vi "traceFileIO_readFromFile.vi"(0 "reference":refnum<class "OSA.lvclass">, 1 "path":path, 3 "dataType":T1, 4 "trace idx":u32, 5 "error in (no error)":errorcluster, 7 "dialog (empty path)":bool) -> (14 "duplicate reference":refnum<class "OSA.lvclass">, 17 "cancelled":bool, 19 "error out":errorcluster)   [LabVIEW 2010, in "OSA.lvclass"]
doc: "Reads trace data from spf2 binary file and store into trace buffer."
uses:
  OSA.lvclass
  typeDef/trace_properties_ui.ctl
  typeDef/acq_dataType.ctl
  OSA20X_misc.lvlib
  FTSLib.dll
panel:
  in  "property":T2=enum."type"
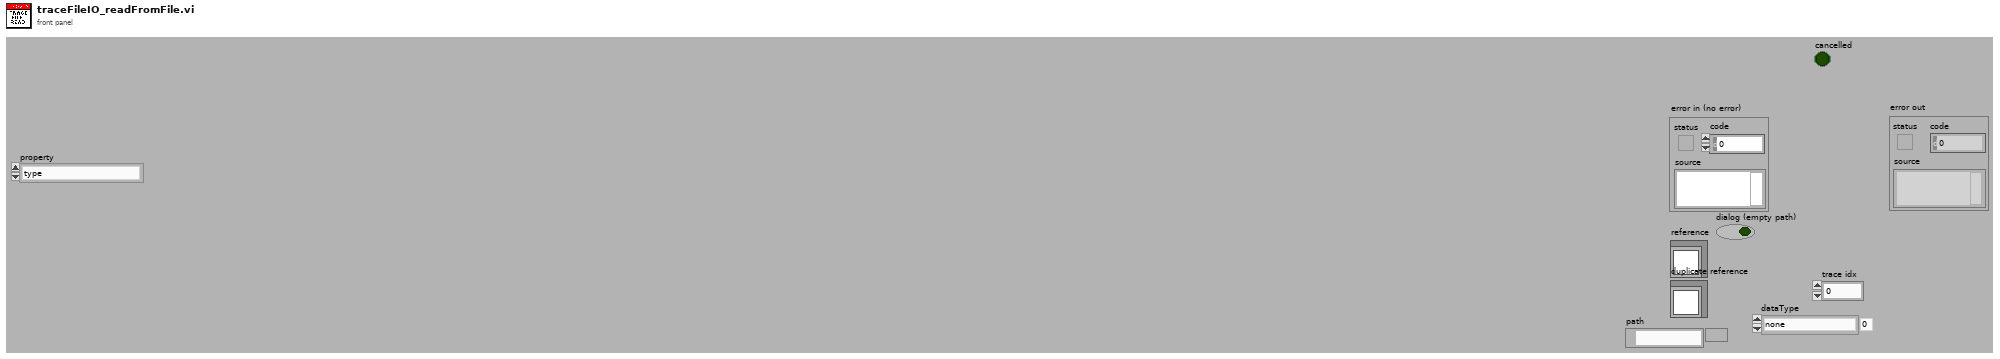
[diagram p1: front panel]
types:
  T1 = typedef "OSA.lvclass/acq_dataType.ctl" = enum16{"none", "interferogram", "spectrum"}
  T2 = typedef "OSA.lvclass/trace_properties_ui.ctl" = enum16{"length", "type", "acquisitionMode", "xValueFormat", "date", "time", "averageNum", "smoothType", "igramSmoothType", "phaseCorrection", "apodisation", "__allocatedLengthI", "__allocatedLengthx", "adcBits", "sensitivityMode", "resolutionMode", "rollingAverage", "samplesPerReference", "air_measureOption", "interferogramProperty", "all_uiProperties"}
  T3 = enum16{"length", "type", "acquisitionMode", "xValueFormat", "date", "time", "averageNum", "smoothType", "igramSmoothType", "phaseCorrection", "apodisation", "__allocatedLengthI", "__allocatedLengthx", "adcBits", "sensitivityMode", "resolutionMode", "rollingAverage", "samplesPerReference", "air_measureOption", "interferogramProperty", "all_uiProperties"}
  T4 = typedef "OSA.lvclass/ObjectAttributes.ctl" = cluster{"Stop":bool, "dataType":T1, "spectrometerIdx":u16, "buffer size interferogram":i32, "interferogram":cluster{"new":bool, "plot_x_ min":sgl, "plot_x_max":sgl, "plot_y_min":sgl, "plot_y_max":sgl, "Graph Intrfrgrm":T5, "timeStamp":u32, "signal (%)":dbl, "traces":cluster{"idx":u32, "broadBand":bool, "monoChromatic":bool, "peakToPeakSignal":dbl, "peakToPeakPos":dbl}[], "traces idx last":i32}, "spectrum":cluster{"new":bool, "plot_x_min":sgl, "plot_x_max":sgl, "plot_unit_x":T6, "plot_unit_y":T7, "plot_y_min":sgl, "plot_y_max":sgl, "Graph Spectrum":T5, "timeStamp":u32, "X_VAL_OPTIONS":enum16{"MIN_MAX", "ARRAY"}, "traces":cluster{"idx":u32}[], "traces idx last":i32}, "Thorlabs_OSA_64.lvclass:queue_action.ctlqueue ref":refnum<queue>, "action":T8, "plot zoom step":dbl, "buffer semaphore":T9, "acq stopped":bool, "dataType active":T1, "temperature (degr C)":sgl, "pressure (hPa)":sgl, "rel humidity (%)":sgl, "settings":cluster{"resolution":u16, "sensitivity":u16, "Average":bool, "average nr":u32, "apodisation":T10, "acq delay (ms)":u32, "airMesure":T11, "wmtr on":bool, "intfgrm_smooth_width":u16, "intfgrm_smooth_nrOfPasses":u16, "intfgrm_smooth":T12, "phaseCorrection":T13, "zeroFill":u8, "spectr_smooth":T12, "spectr_smooth_width":u16, "spectr_smooth_nrOfPasses":u16, "resolution (/cm)":sgl, "REF wavelength, (nm)":dbl, "gain_idx":u16, "gainAuto":bool, "gain_relative":dbl, "PD sensitivity mode":T14, "PD senseMode implemented":bool, "SensorTemperature implemented":bool, "SensorPressure implemented":bool, "SensorHumidity implemented":bool}, "peaks position":sgl[], "peaks width":sgl[], "peaks height":sgl[], "peaks max nr":u32, "peaks latest nr":i32, "peaks new":bool, "power":dbl, "power new":bool, "path":string, "wavelength (WNr)":dbl, "wavelength new":bool, "buffer size spectrum":i32, "status":string, "VI reference":refnum<vi>, "funcPointer":u64, "libraryPointer":u64, "singleAcquisition":bool, "coherenceLength (cm)":dbl, "coherenceLength new":bool, "spectrometer model":string, "spectrometer serial nr":string, "peaks thld left":sgl[], "peaks thld right":sgl[], "coherenceLength error (cm)":dbl, "ADC bits":u16, "peaks position centroid":sgl[], "peaks height centroid":sgl[], "OSA series":T15, "channel index spectrum":u16, "spectrometer rangeLow, (/cm)":dbl, "spectrometer rangeHigh, (/cm)":dbl, "channel index interferogram":u16}
  T5 = typedef "OSA.lvclass/graph_intensity.ctl" = refnum<vi>
  T6 = typedef "OSA.lvclass/spectrum_x_unit.ctl" = enum16{"wavenr/cm", "THz", "eV", "nm_air", "nm_vac"}
  T7 = typedef "OSA.lvclass/y_unit.ctl" = enum16{"ADC counts", "dBm pwr absolute", "dBm pwr density", "mW pwr absolute", "mW pwr density"}
  T8 = typedef "OSA.lvclass/queue_action.ctl" = enum16{"none", "stop", "GUI_plotInterferogram", "GUI_plotSpectrum", "GUI_plotInterferogramRescale", "GUI_plotSpectrumRescale", "GUI_plotInterferogramReset", "GUI_plotSpectrumReset", "GUI_plotInterferogramAutoScaleY", "GUI_plotSpectrumAutoScaleY", "GUI_plotInterferogramZoomOut", "GUI_plotSpectrumZoomOut", "GUI_plotInterferogramPane", "GUI_plotSpectrumPane", "GUI_plotInterferogramZoomMouse", "GUI_plotSpectrumZoomMouse", "ENVIRONMENT temperature", "ENVIRONMENT pressure", "MODE_resolution set", "MODE_resolution get", "MODE_sensitivity set", "MODE_sensitivity get", "MODE_PDTemperature set", "MODE_PDTemperature get", "REBOOT/RESET firmware", "ACQASYNC_acquireSingleSpectrum", "ACQASYNC_continuous start", "ACQASYNC_continuous stop\n", "ACQASYNC_get last interferogram", "ACQASYNC_get last spectrum", "ACQASYNC_get last waveNr", "ACQOPT_interferogram smoothing set", "ACQOPT_interferogram smoothing get", "ACQOPT_spectrum smoothing set", "ACQOPT_spectrum smoothing get", "ACQOPT_apodisation type set", "ACQOPT_apodisation type get", "ACQOPT_phase correction type set", "ACQOPT_phase correction type get", "ACQOPT_acqIntervall_set", "ACQOPT_acqIntervall_get", "ACQOPT_average spectrum set", "ACQOPT_average spectrum get", "ACQOPT_rolling average set", "ACQOPT_rolling average get", "ACQOPT_zero fill factor set", "ACQOPT_zero fill factor get", "ACQOPT_cycle counting set", "ACQOPT_cycle counting get", "ACQOPT_air measure option set", "ACQOPT_air measure option get", "ACQOPT_gainLevel auto get", "ACQOPT_gainLevel auto set", "ACQOPT_gainLevel get", "ACQOPT_gainLevel set", "ACQOPT_getAll", "INSTRUMENT_PROPERTY_range_WaveNr_min", "INSTRUMENT_PROPERTY_range_WaveNr_max", "INSTRUMENT_PROPERTY_reference_wavelength_cm^-1", "INSTRUMENT_PROPERTY_samplesPerRefPeriod", "INSTRUMENT_PROPERTY_resolution_waveNrPercm", "INSTRUMENT_PROPERTY_availableGainLevels", "INSTRUMENT_PROPERTY_status", "CONVERT", "ANALYSE_POWER", "ANALYSE_PEAKS", "ANALYSE_WAVELENGTH", "ANALYSE_SPECTRUM", "ANALYSE_INTERFEROGRAM", "ANALYSE_COHERENCE_LENGTH", "MATH", "MATH_power", "MATH_peaks", "FILE", "miscellaneous"}
  T9 = typedef "Semaphore RefNum" = refnum<k1>
  T10 = typedef "OSA.lvclass/apodisation.ctl" = enum16{"NONE", "NORTON_BEER_WEAK", "NORTON_BEER_MEDIUM", "NORTON_BEER_STRONG", "TRIANGULAR", "COSINE", "HANN", "HAMMING", "BLACKMANHARRIS3", "BLACKMANHARRIS4", "GAUSSIAN"}
  T11 = typedef "OSA.lvclass/airMeasure.ctl" = enum16{"TEMPERATURE", "PRESSURE"}
  T12 = typedef "OSA20X_misc.lvlib/interferogram_smoothing.ctl" = enum16{"NONE", "BINOMIAL", "SAVITSKY_GOLAY", "FOURIER", "MOVING_AVERAGE", "GAUSSIAN"}
  T13 = typedef "OSA.lvclass/phaseCorrection.ctl" = enum16{"NONE", "MERTZ", "FORMAN", "MERTZ_FILE", "FORMAN_FILE", "FUTURE COMP."}
  T14 = typedef "OSA20X_misc.lvlib/PDTemperatureMode.ctl" = enum16{"cool: better sensitivity/noise floor", "warm: extended wl range"}
  T15 = typedef "OSA.lvclass/OSA_series.ctl" = enum16{"OSA200", "OSA300", "UNKNOWN"}
  T16 = cluster{"idx":u32, "broadBand":bool, "monoChromatic":bool, "peakToPeakSignal":dbl, "peakToPeakPos":dbl}[]
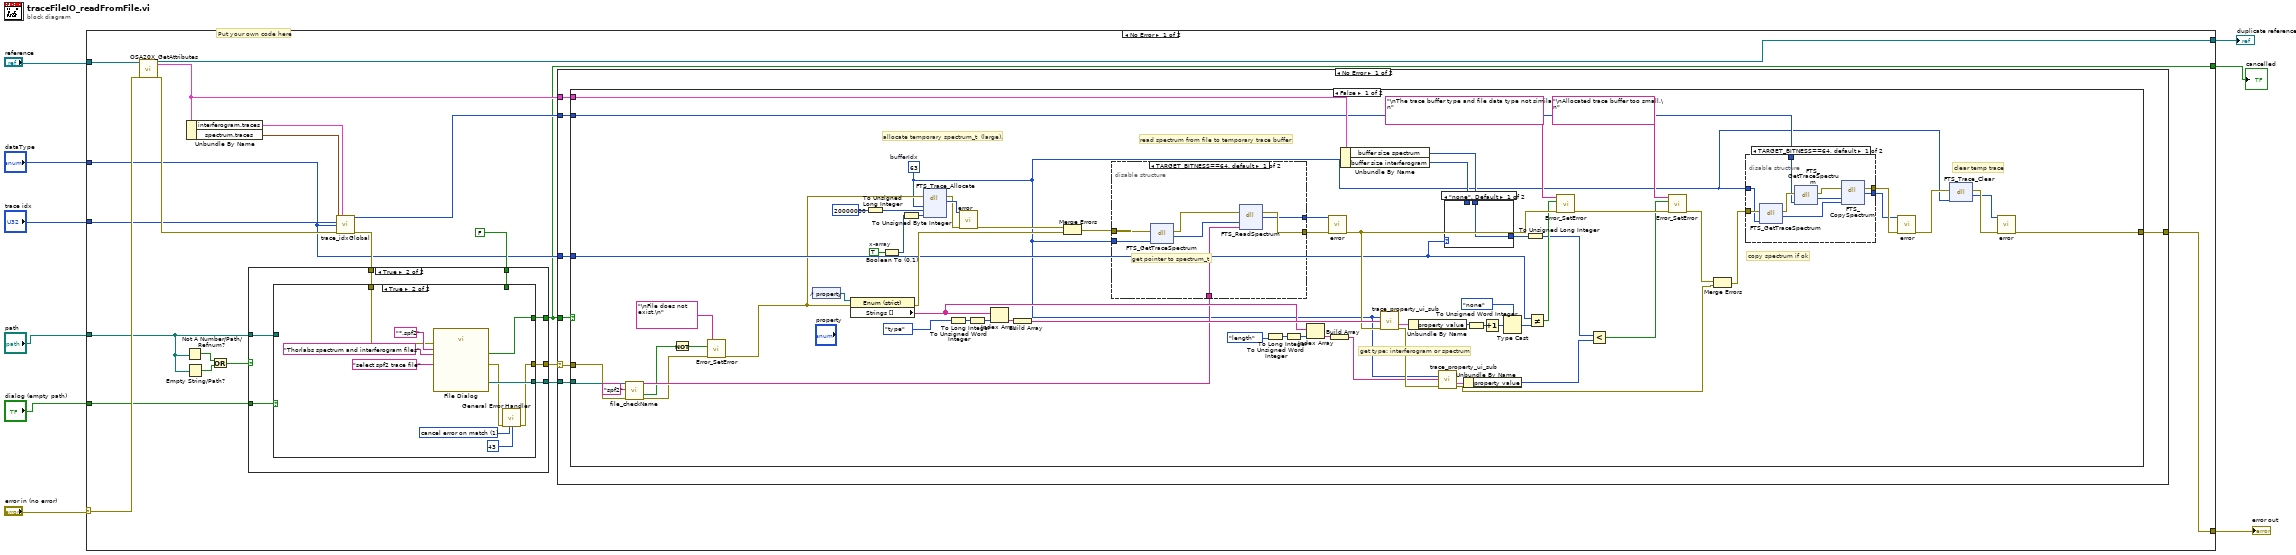
[diagram p0: block diagram]
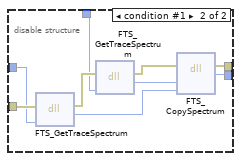
[diagram p2: hidden frame]
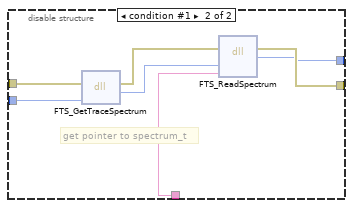
[diagram p4: hidden frame]
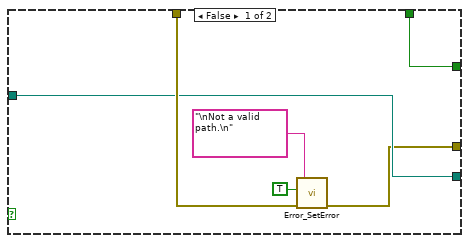
[diagram p8: hidden frame]
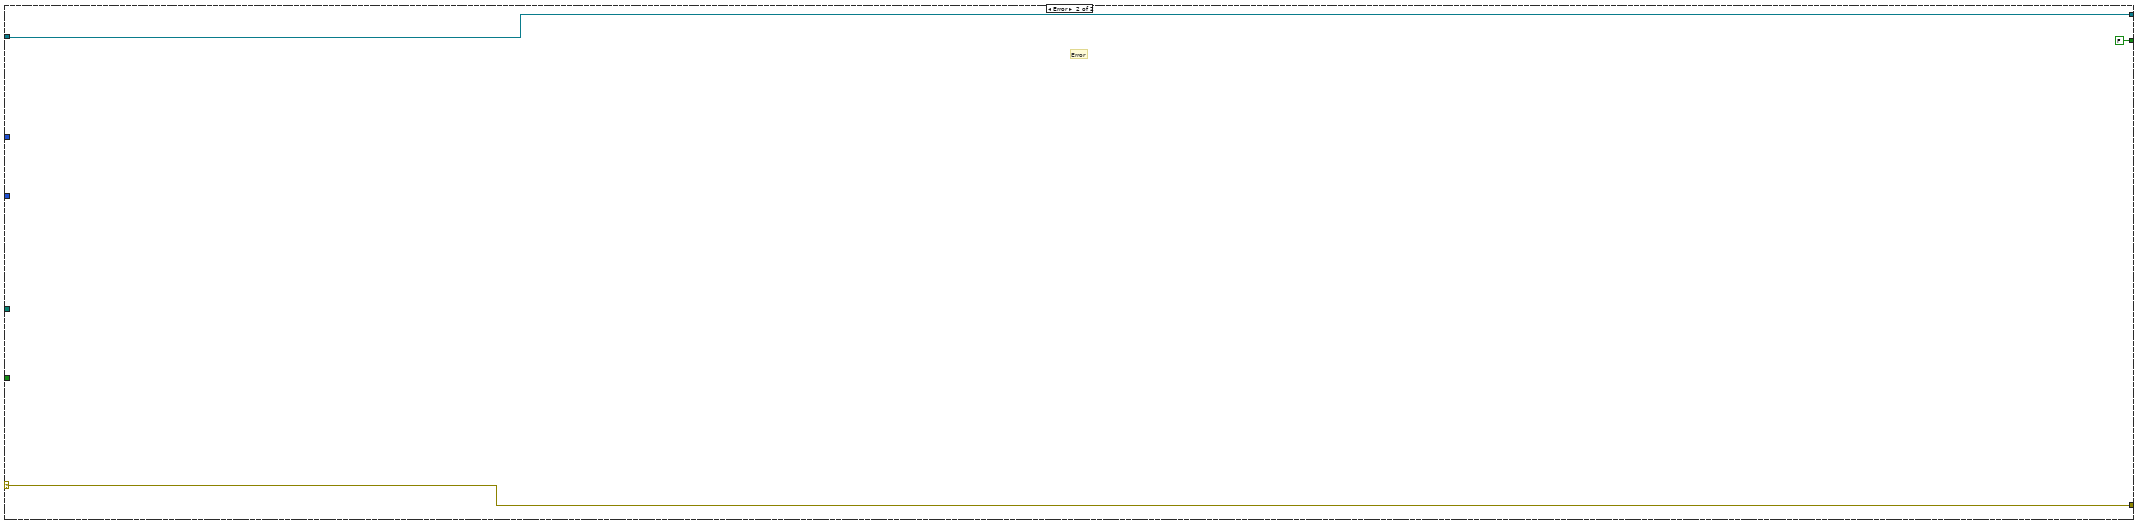
[diagram p9: hidden frame]
diagram:
  n1 = case shown="No Error" "error in (no error)" {
    selector: "error in (no error)" -> [w29 w167]
    tunnel: [w19 w167] -> w8
    tunnel: "reference" -> [w30 w166]
    tunnel: [w20 w166] -> w6
    tunnel: "trace idx" -> [w13 _]
    tunnel: "path" -> [w14 _]
    tunnel: "dataType" -> [w12 _]
    tunnel: "dialog (empty path)" -> [w11 _]
    tunnel: [w10 FALSE ("cancelled")] -> w1
    frame No Error {
      # "Put your own code here"
      n2 = call "OSA20X_GetAttributes.vi"("reference in"=w30, "error in (no error)"=w29) -> ("reference out"=w20:refnum<class "OSA.lvclass">, "Data"=w16:T4, "error out"=w15:errorcluster)  [unwired: 14 in, 1 out]
      n3 = Not A Number/Path/Refnum?(number/path/refnum=w14) -> (NaN/Path/Refnum?=w27:bool)
      n4 = Empty String/Path?(string/path=w14) -> (empty?=w28:bool)
      n5 = Unbundle By Name(w16) -> ("interferogram.traces"=w18:T16, "spectrum.traces"=w17:cluster{"idx":u32}[])
      n6 = Or(x=w27, y=w28) -> (x .or. y?=w26:bool)
      n7 = call "trace_idxGlobal.vi"("traces_spectrum"=w17, "traces_interferogram"=w18, "trace idx"=w13, "dataType"=w12, "error in (no error)"=w15) -> ("global trace idx"=w25:u32, "error out"=w24:errorcluster)  [unwired: 9 in]
      n8 = case shown="True" w26 {
        tunnel: w14 -> [w140 w144]
        tunnel: w11 -> [_ w148]
        tunnel: w24 -> [w141 w147]
        tunnel: [w139 w145] -> w10
        tunnel: [w140 w146] -> w22
        tunnel: [w141 w143] -> w23
        tunnel: FALSE ("cancelled") -> [w139 w142]
        frame False {
        }
        frame True {
          n9 = case shown="True" w148 {
            tunnel: w147 -> [w154 w161]
            tunnel: [w151 w160] -> w146
            tunnel: [w149 w159] -> w145
            tunnel: w144 -> [w151 _]
            tunnel: [w150 w155] -> w143
            tunnel: w142 -> [w149 _]
            frame False {
              n10 = call "Error_SetError.vi"("error in"=w154, "status (true)"=TRUE, "source(\"\")"="\nNot a valid path.\n" ("source(\"\")")) -> ("error out"=w150:errorcluster)  [unwired: 4 in]
            }
            frame True {
              w158 = 1 items=["no exception", "cancel error on match", "set error on match"] ("[exception action] (none:0)")
              n11 = call "File Dialog"("prompt"="select spf2 trace file", "error in"=w161, "pattern (all files)"="*.spf2", "pattern label"="Thorlabs spectrum and interferogram files") -> ("selected path"=w160:path, "cancelled"=w159:bool, "error out"=w156:errorcluster)  [unwired: 8 in, 1 out]
              n12 = call <vilib>:"General Error Handler.vi"("error in (no error)"=w156, "[exception action] (none:0)"=w158, "[exception code]"=43) -> ("error out"=w155:errorcluster)  [unwired: 8 in, 4 out]
            }
          }
        }
      }
      n13 = case shown="No Error" w23 {
        selector: w23 -> [w35 w138]
        tunnel: w25 -> [w37 _]
        tunnel: [w36 w138] -> w19
        tunnel: w10 -> [w33 _]
        tunnel: w22 -> [w34 _]
        tunnel: w12 -> [w32 _]
        tunnel: w16 -> [w31 _]
        frame No Error {
          n14 = case shown="False" w33 {
            tunnel: w37 -> [w57 _]
            tunnel: [w39 w137] -> w36
            tunnel: w35 -> [w51 w137]
            tunnel: w34 -> [w50 _]
            tunnel: w32 -> [w63 _]
            tunnel: w31 -> [w68 _]
            frame False {
              w100 = TRUE  # x-array
              w41 = u32 63  # bufferIdx
              # "clear temp trace"
              # "copy spectrum if ok"
              # "get type: interferogram or spectrum"
              # "read spectrum from file to temporary trace buffer"
              # "allocate temporary spectrum_t  (large)."
              n15 = call "file_checkName.vi"("path"=w50, "filename extension"="spf2", "error in (no error)"=w51) -> ("path string out"=w48:string, "exist"=w44:bool, "error out"=w46:errorcluster)  [unwired: 13 in, 1 out]
              n16 = Not(x=w44) -> (.not. x?=w43:bool)
              n17 = call "Error_SetError.vi"("error in"=w46, "status (true)"=w43, "source(\"\")"="\nFile does not exist.\n" ("source(\"\")")) -> ("error out"=w45:errorcluster)  [unwired: 4 in]
              n18 = control-ref of="property"() -> (w95:refnum<vi>)
              n19 = property class="Enum (strict)"(reference=w95, error in=w45) -> (error out=w88:errorcluster, "Strings []"=w72:string[])  [unwired: 1 out]
              n20 = To Unsigned Long Integer(number=u32 20000000) -> (unsigned 32bit integer=w101:u32)
              n21 = Boolean To (0,1)(Boolean=w100) -> (0, 1=w99:i16)
              n22 = To Unsigned Byte Integer(number=w99) -> (unsigned 8bit integer=w98:u8)
              n23 = dll-call lib="FTSLib.dll" fn="FTS_Trace_Allocate"(error in=w45, "bufferIdx"=w41, "spectrumLength"=w101, "addX"=w98) -> (error out=w96:errorcluster, "returnValue"=w97:i32)  [unwired: 5 in, 1 out]
              n24 = To Unsigned Word Integer(number=T3."type" ("Value")) -> (unsigned 16bit integer=w94:u16)
              n25 = call "error.vi"("result code"=w97, "error in (no error)"=w96) -> ("error out"=w89:errorcluster)  [unwired: 15 in, 2 out]
              n26 = To Long Integer(number=w94) -> (32bit integer=w93:i32)
              n27 = Index Array(array=w72, index=w93) -> (element=w92:string)
              n28 = Build Array(w92) -> (w91:string[])
              n29 = Merge Errors(w89, w88) -> (w87:errorcluster)
              n30 = disable-structure shown="TARGET_BITNESS==64, default" {
                disable-tunnel: w41 -> [w124 w133]
                disable-tunnel: w48 -> [w129 w132]
                disable-tunnel: w87 -> [w127 w134]
                disable-tunnel: [w126 w131] -> w102
                disable-tunnel: [w125 w130] -> w90
                frame condition #0 (active) {
                  # "get pointer to spectrum_t"
                  n31 = dll-call lib="FTSLib.dll" fn="FTS_GetTraceSpectrum"(error in=w127, "traceIdx"=w124) -> (error out=w128:errorcluster, "spectrum_t_pointer"=w123:u64)  [unwired: 3 in, 1 out]
                  n32 = dll-call lib="FTSLib.dll" fn="FTS_ReadSpectrum"(error in=w128, "spectrum_t_pointer"=w123, "fileNameAndPath"=w129) -> (error out=w126:errorcluster, "returnValue"=w125:i32)  [unwired: 4 in, 1 out]
                }
                frame condition #1 {
                  # "get pointer to spectrum_t"
                  n33 = dll-call lib="FTSLib.dll" fn="FTS_GetTraceSpectrum"(error in=w134, "traceIdx"=w133) -> (error out=w135:errorcluster, "spectrum_t_pointer"=w136:u32)  [unwired: 3 in, 1 out]
                  n34 = dll-call lib="FTSLib.dll" fn="FTS_ReadSpectrum"(error in=w135, "spectrum_t_pointer"=w136, "fileNameAndPath"=w132) -> (error out=w131:errorcluster, "parameter"=w130:i32)  [unwired: 4 in, 1 out]
                }
              }
              n35 = To Unsigned Word Integer(number=T3."length" ("Value")) -> (unsigned 16bit integer=w76:u16)
              n36 = To Long Integer(number=w76) -> (32bit integer=w75:i32)
              n37 = Index Array(array=w72, index=w75) -> (element=w74:string)
              n38 = call "error.vi"("result code"=w90, "error in (no error)"=w102) -> ("error out"=w81:errorcluster)  [unwired: 15 in, 2 out]
              n39 = Build Array(w74) -> (w71:string[])
              n40 = Unbundle By Name(w68) -> ("buffer size spectrum"=w61:i32, "buffer size interferogram"=w62:i32)
              n41 = call "trace_property_ui_sub.vi"("trace idx global"=w41, "properties ui"=w91, "error in (no error)"=w81) -> ("property"=w86:cluster{"property":string, "property value":u32}, "error out"=w78:errorcluster)  [unwired: 10 in, 1 out]
              n42 = Unbundle By Name(w86) -> ("property value"=w85:u32)
              n43 = call "trace_property_ui_sub.vi"("trace idx global"=w41, "properties ui"=w71, "error in (no error)"=w78) -> ("property"=w70:cluster{"property":string, "property value":u32}, "error out"=w53:errorcluster)  [unwired: 10 in, 1 out]
              n44 = case shown="\"none\", Default" w63 {
                tunnel: w62 -> [_ w122]
                tunnel: w61 -> [w121 _]
                tunnel: [w121 w122] -> w60
                frame "none", Default {
                }
                frame "interferogram" {
                }
              }
              n45 = Unbundle By Name(w70) -> ("property value"=w67:u32)
              n46 = To Unsigned Word Integer(number=w85) -> (unsigned 16bit integer=w83:u16)
              n47 = Increment(x=w83) -> (x+1=w82:u16)
              n48 = Type Cast(type=acq_dataType."none" ("dataType"), x=w82) -> (*(type *) &x=w69:T1)
              n49 = To Unsigned Long Integer(number=w60) -> (unsigned 32bit integer=w59:u32)
              n50 = Not Equal?(x=w63, y=w69) -> (x != y?=w80:bool)
              n51 = call "Error_SetError.vi"("error in"=w81, "status (true)"=w80, "source(\"\")"="\nThe trace buffer type and file data type not similar.\n" ("source(\"\")")) -> ("error out"=w66:errorcluster)  [unwired: 4 in]
              n52 = Less?(x=w59, y=w67) -> (x < y?=w58:bool)
              n53 = call "Error_SetError.vi"("error in"=w66, "status (true)"=w58, "source(\"\")"="\nAllocated trace buffer too small.\n" ("source(\"\")")) -> ("error out"=w54:errorcluster)  [unwired: 4 in]
              n54 = Merge Errors(w54, w53) -> (w52:errorcluster)
              n55 = disable-structure shown="TARGET_BITNESS==64, default" {
                disable-tunnel: w52 -> [w109 w116]
                disable-tunnel: [w106 w114] -> w56
                disable-tunnel: [w105 w113] -> w55
                disable-tunnel: w41 -> [w104 w115]
                disable-tunnel: w57 -> [w103 w112]
                frame condition #0 (active) {
                  n56 = dll-call lib="FTSLib.dll" fn="FTS_GetTraceSpectrum"(error in=w109, "traceIdx"=w104) -> (error out=w108:errorcluster, "spectrum_t_pointer"=w110:u64)  [unwired: 3 in, 1 out]
                  n57 = dll-call lib="FTSLib.dll" fn="FTS_GetTraceSpectrum"(error in=w108, "traceIdx"=w103) -> (error out=w107:errorcluster, "spectrum_t_pointer"=w111:u64)  [unwired: 3 in, 1 out]
                  n58 = dll-call lib="FTSLib.dll" fn="FTS_CopySpectrum"(error in=w107, "spectrum_t_pointer_to"=w111, "spectrum_t_pointer_from"=w110) -> (error out=w106:errorcluster, "returnValue"=w105:i32)  [unwired: 4 in, 1 out]
                }
                frame condition #1 {
                  n59 = dll-call lib="FTSLib.dll" fn="FTS_GetTraceSpectrum"(error in=w116, "traceIdx"=w115) -> (error out=w118:errorcluster, "spectrum_t_pointer"=w119:u32)  [unwired: 3 in, 1 out]
                  n60 = dll-call lib="FTSLib.dll" fn="FTS_GetTraceSpectrum"(error in=w118, "traceIdx"=w112) -> (error out=w117:errorcluster, "spectrum_t_pointer"=w120:u32)  [unwired: 3 in, 1 out]
                  n61 = dll-call lib="FTSLib.dll" fn="FTS_CopySpectrum"(error in=w117, "spectrum_t_pointer_to"=w120, "spectrum_t_pointer_from"=w119) -> (error out=w114:errorcluster, "returnValue"=w113:i32)  [unwired: 4 in, 1 out]
                }
              }
              n62 = call "error.vi"("result code"=w55, "error in (no error)"=w56) -> ("error out"=w42:errorcluster)  [unwired: 15 in, 2 out]
              n63 = dll-call lib="FTSLib.dll" fn="FTS_Trace_Clear"(error in=w42, "bufferIdx"=w41) -> (error out=w40:errorcluster, "returnValue"=w38:i32)  [unwired: 3 in, 1 out]
              n64 = call "error.vi"("result code"=w38, "error in (no error)"=w40) -> ("error out"=w39:errorcluster)  [unwired: 15 in, 2 out]
            }
            frame True {
            }
          }
        }
        frame Error {
        }
      }
    }
    frame Error {
      # "Error"
    }
  }
  "error out" <- w8
  "duplicate reference" <- w6
  "cancelled" <- w1
